vi "前面板对象数据传递.vi"() -> ()   [LabVIEW 2010]
uses:
  <vilib>/Analysis/NI_AALBase.lvlib
panel:
  in  "停止":bool
  in  "幅度显示":u8(slide)=3 scale=0.0..10.0
  out "波形显示":dbl[](graph)
  # "1.按照教材要求修改各个控件链接的URL\n2.打开DataSocket Server\n3.运行此VI\n4.运行前面板对象数据接收VI"
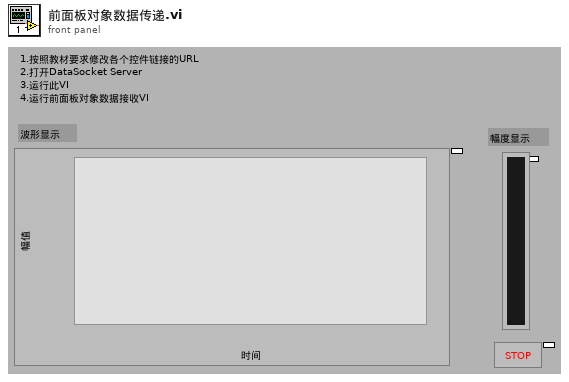
[diagram p1: front panel]
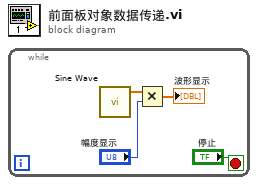
[diagram p0: block diagram]
diagram:
  n1 = while {
    stop <- "停止" stop-if-true
    n2 = call <vilib>:"Sine Wave.vi"() -> ("sine wave"=w4:dbl[])  [unwired: 5 in, 2 out]
    n3 = Multiply(x=w4, y="幅度显示") -> (x*y=→"波形显示":dbl[])
  }
